vi "Create.vi"() -> (8 "FSM.Annotation":refnum<class "FSM.Annotation.lvclass">)   [LabVIEW 2020, in "FSM.Annotation.lvclass"]
uses:
  FSM.Annotation.lvclass
  FSM.Annotation.lvclass/FSM.Annotation.ctl
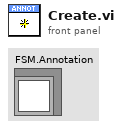
[diagram p1: front panel]
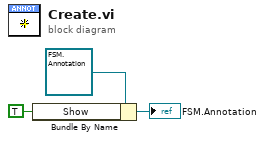
[diagram p0: block diagram]
diagram:
  n1 = Bundle By Name(cluster=refnum<class "FSM.Annotation.lvclass"> refnum ("FSM.Annotation"), "Show"=TRUE ("Serialized.Show")) -> (→"FSM.Annotation":refnum<class "FSM.Annotation.lvclass">)
